vi "Control Panel Values Changed.vi"(8 "error in (no error)":errorcluster, 9 "Old data":variant, 10 "New data":variant, 11 "Device in":refnum<class "Cryo-Con-22C.lvclass">) -> (0 "error out":errorcluster, 3 "Device out":refnum<class "Cryo-Con-22C.lvclass">)   [LabVIEW 2015, in "Cryo-Con-22C.lvclass"]
uses:
  Cryo-Con-22C.lvclass
  Cryo-Con Front Panel Data.ctl
  Cryo-con Heater Ranges.ctl
  Cry-Con Loop Type.ctl
  Instrument/Read VISA Resource.vi
  Instrument/Write VISA Resource.vi
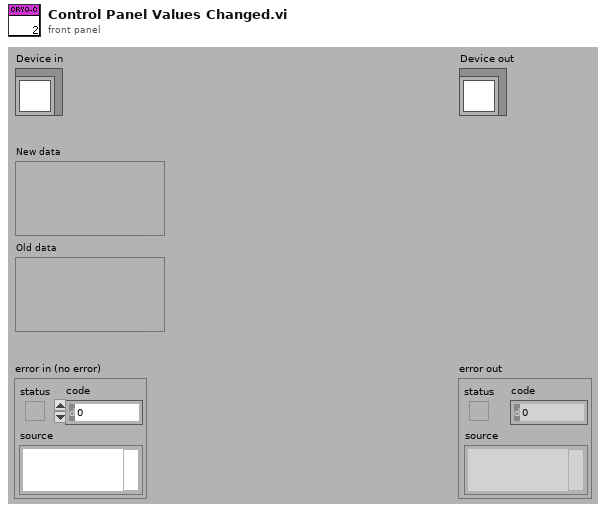
[diagram p1: front panel]
types:
  T1 = typedef "Cryo-Con Front Panel Data.ctl" = cluster{"Channels to measure":string[], "Record heater":bool, "Set point":dbl, "Heater Range":T2, "Control":bool, "Loop type":T3, "Ramp rate,\n K/min":dbl, "Control Channel":string, "P":dbl, "I":dbl, "D":dbl, "Manual %":u16}
  T2 = typedef "Cryo-con Heater Ranges.ctl" = enum16{"25W", "2.5W", "0.25W"}
  T3 = typedef "Cry-Con Loop Type.ctl" = enum16{"Off", "PID", "Manual", "PID Table", "PID Ramp", "PID Table Ramp"}
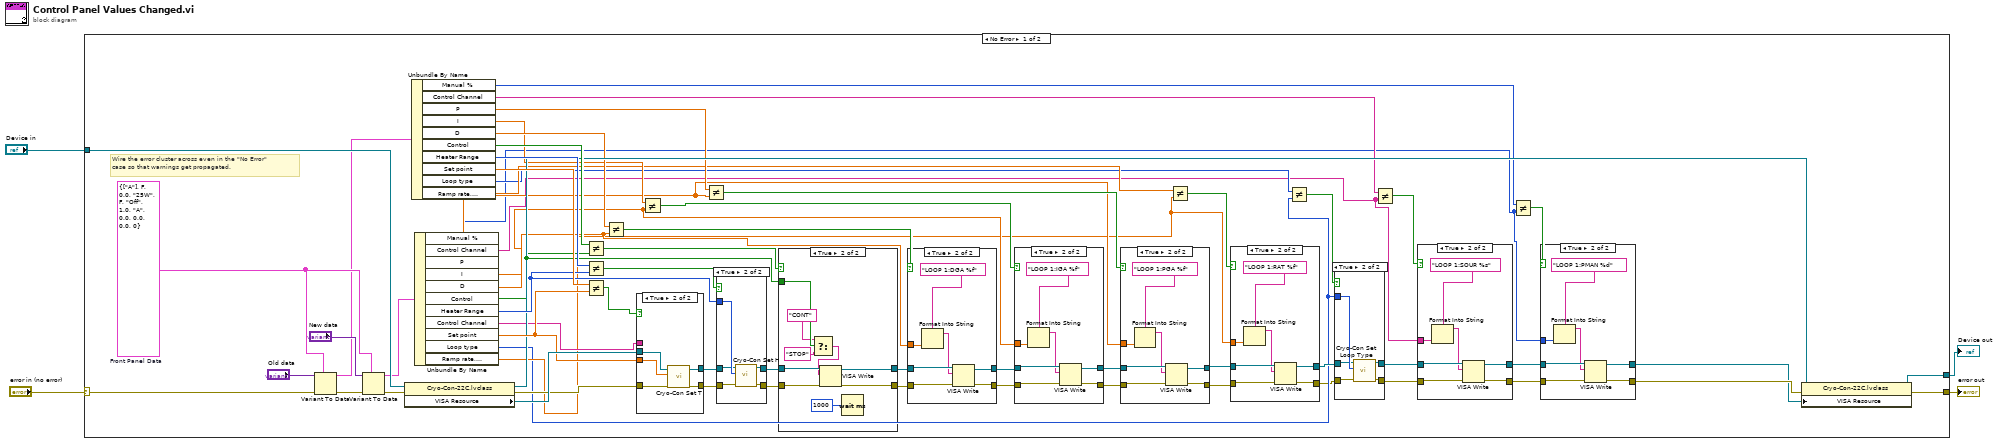
[diagram p0: block diagram]
diagram:
  n1 = case shown="No Error" "error in (no error)" {
    selector: "error in (no error)" -> [w69 w157]
    tunnel: [w66 w157] -> w3
    tunnel: [w67 w156] -> w1
    tunnel: "Device in" -> [w68 w156]
    frame No Error {
      w64 = T1 {"Channels to measure"=["A"], "Record heater"=FALSE, "Set point"=0.0, "Heater Range"=enum."25W", "Control"=FALSE, "Loop type"=enum."Off", "Ramp rate,\n K/min"=1.0, "Control Channel"="A", "P"=0.0, "I"=0.0, "D"=0.0, "Manual %"=0}  # Front Panel Data
      # "Wire the error cluster across even in the \"No Error\"\ncase so that warnings get propagated."
      n2 = Variant To Data(error in=w69, type=w64, Variant="Old data") -> (data=w44:T1, error out=w65:errorcluster)
      n3 = Variant To Data(error in=w65, type=w64, Variant="New data") -> (data=w45:T1, error out=w61:errorcluster)
      n4 = property class="Cryo-Con-22C.lvclass"(reference=w68, error in=w61) -> (reference out=w47:refnum<class "Cryo-Con-22C.lvclass">, error out=w60:errorcluster, "VISA Resource"=w62:refnum<visa-resource-name>)
      n5 = Unbundle By Name(w44) -> ("Manual %"=w11:u16, "Control Channel"=w16:string, "P"=w29:dbl, "I"=w35:dbl, "D"=w40:dbl, "Control"=w53:bool, "Heater Range"=w58:T2, "Set point"=w63:dbl, "Loop type"=w20:T3, "Ramp rate,\n K/min"=w26:dbl)
      n6 = Unbundle By Name(w45) -> ("Manual %"=w9:u16, "Control Channel"=w14:string, "P"=w28:dbl, "I"=w33:dbl, "D"=w38:dbl, "Control"=w41:bool, "Heater Range"=w48:T2, "Control Channel"=w46:string, "Set point"=w49:dbl, "Loop type"=w18:T3, "Ramp rate,\n K/min"=w24:dbl)
      n7 = Not Equal?(x=w53, y=w41) -> (x != y?=w55:bool)
      n8 = Not Equal?(x=w58, y=w48) -> (x != y?=w59:bool)
      n9 = Not Equal?(x=w63, y=w49) -> (x != y?=w27:bool)
      n10 = Not Equal?(x=w40, y=w38) -> (x != y?=w39:bool)
      n11 = case shown="True" w27 {
        tunnel: w60 -> [w150 w155]
        tunnel: [w150 w154] -> w57
        tunnel: w49 -> [_ w151]
        tunnel: w62 -> [w149 w152]
        tunnel: [w149 w153] -> w56
        tunnel: w46 -> [_ _]
        frame False {
        }
        frame True {
          n12 = call "Cryo-Con Set T.vi"("error in (no error)"=w155, "Set T"=w151, "VISA Resource Name"=w152) -> ("error out"=w154:errorcluster, "VISA Resource Name Out"=w153:refnum<visa-resource-name>)  [unwired: 7 in]
        }
      }
      n13 = Not Equal?(x=w35, y=w33) -> (x != y?=w34:bool)
      n14 = Not Equal?(x=w29, y=w28) -> (x != y?=w30:bool)
      n15 = case shown="True" w59 {
        tunnel: w57 -> [w143 w146]
        tunnel: [w143 w145] -> w54
        tunnel: w48 -> [_ w148]
        tunnel: [w142 w144] -> w52
        tunnel: w56 -> [w142 w147]
        frame False {
        }
        frame True {
          n16 = call "Cryo-Con Set H.vi"("error in (no error)"=w146, "Set T"=w148, "VISA Resource Name"=w147) -> ("error out"=w145:errorcluster, "VISA Resource Name Out"=w144:refnum<visa-resource-name>)  [unwired: 7 in]
        }
      }
      n17 = case shown="True" w55 {
        tunnel: w54 -> [w132 w139]
        tunnel: [w132 w141] -> w42
        tunnel: w41 -> [_ w137]
        tunnel: [w131 w138] -> w43
        tunnel: w52 -> [w131 w140]
        frame False {
        }
        frame True {
          n18 = Select(t="CONT", s=w137, f="STOP") -> (s? t:f=w134:string)
          n19 = VISA Write(VISA resource name=w140, write buffer=w134, error in (no error)=w139) -> (VISA resource name out=w138:refnum<visa-resource-name>, error out=w141:errorcluster)  [unwired: 1 out]
          n20 = Wait (ms)(milliseconds to wait=u32 1000) -> ()  [unwired: 1 out]
        }
      }
      n21 = case shown="True" w39 {
        tunnel: w42 -> [w123 w128]
        tunnel: [w123 w130] -> w36
        tunnel: w38 -> [_ w126]
        tunnel: [w122 w127] -> w37
        tunnel: w43 -> [w122 w129]
        frame False {
        }
        frame True {
          n22 = Format Into String(format string="LOOP 1:DGA %f", w126) -> (resulting string=w124:string)  [unwired: 2 in, 1 out]
          n23 = VISA Write(VISA resource name=w129, write buffer=w124, error in (no error)=w128) -> (VISA resource name out=w127:refnum<visa-resource-name>, error out=w130:errorcluster)  [unwired: 1 out]
        }
      }
      n24 = case shown="True" w34 {
        tunnel: w36 -> [w114 w119]
        tunnel: [w114 w121] -> w31
        tunnel: w33 -> [_ w117]
        tunnel: [w113 w118] -> w32
        tunnel: w37 -> [w113 w120]
        frame False {
        }
        frame True {
          n25 = Format Into String(format string="LOOP 1:IGA %f", w117) -> (resulting string=w115:string)  [unwired: 2 in, 1 out]
          n26 = VISA Write(VISA resource name=w120, write buffer=w115, error in (no error)=w119) -> (VISA resource name out=w118:refnum<visa-resource-name>, error out=w121:errorcluster)  [unwired: 1 out]
        }
      }
      n27 = case shown="True" w30 {
        tunnel: w31 -> [w105 w110]
        tunnel: [w105 w112] -> w23
        tunnel: w28 -> [_ w108]
        tunnel: [w104 w109] -> w22
        tunnel: w32 -> [w104 w111]
        frame False {
        }
        frame True {
          n28 = Format Into String(format string="LOOP 1:PGA %f", w108) -> (resulting string=w106:string)  [unwired: 2 in, 1 out]
          n29 = VISA Write(VISA resource name=w111, write buffer=w106, error in (no error)=w110) -> (VISA resource name out=w109:refnum<visa-resource-name>, error out=w112:errorcluster)  [unwired: 1 out]
        }
      }
      n30 = Not Equal?(x=w26, y=w24) -> (x != y?=w25:bool)
      n31 = case shown="True" w25 {
        tunnel: w23 -> [w96 w101]
        tunnel: [w96 w103] -> w17
        tunnel: w24 -> [_ w99]
        tunnel: [w95 w100] -> w21
        tunnel: w22 -> [w95 w102]
        frame False {
        }
        frame True {
          n32 = Format Into String(format string="LOOP 1:RAT %f", w99) -> (resulting string=w97:string)  [unwired: 2 in, 1 out]
          n33 = VISA Write(VISA resource name=w102, write buffer=w97, error in (no error)=w101) -> (VISA resource name out=w100:refnum<visa-resource-name>, error out=w103:errorcluster)  [unwired: 1 out]
        }
      }
      n34 = Not Equal?(x=w20, y=w18) -> (x != y?=w19:bool)
      n35 = case shown="True" w19 {
        tunnel: w17 -> [w89 w92]
        tunnel: [w89 w91] -> w12
        tunnel: w18 -> [_ w94]
        tunnel: [w88 w90] -> w13
        tunnel: w21 -> [w88 w93]
        frame False {
        }
        frame True {
          n36 = call "Cryo-Con Set Loop Type.vi"("error in (no error)"=w92, "Set T"=w94, "VISA Resource Name"=w93) -> ("error out"=w91:errorcluster, "VISA Resource Name Out"=w90:refnum<visa-resource-name>)  [unwired: 7 in]
        }
      }
      n37 = Not Equal?(x=w16, y=w14) -> (x != y?=w15:bool)
      n38 = case shown="True" w15 {
        tunnel: w12 -> [w80 w85]
        tunnel: [w80 w87] -> w8
        tunnel: w14 -> [_ w83]
        tunnel: [w79 w84] -> w7
        tunnel: w13 -> [w79 w86]
        frame False {
        }
        frame True {
          n39 = Format Into String(format string="LOOP 1:SOUR %s", w83) -> (resulting string=w81:string)  [unwired: 2 in, 1 out]
          n40 = VISA Write(VISA resource name=w86, write buffer=w81, error in (no error)=w85) -> (VISA resource name out=w84:refnum<visa-resource-name>, error out=w87:errorcluster)  [unwired: 1 out]
        }
      }
      n41 = Not Equal?(x=w11, y=w9) -> (x != y?=w10:bool)
      n42 = case shown="True" w10 {
        tunnel: w8 -> [w71 w76]
        tunnel: [w71 w78] -> w6
        tunnel: w9 -> [_ w74]
        tunnel: [w70 w75] -> w5
        tunnel: w7 -> [w70 w77]
        frame False {
        }
        frame True {
          n43 = Format Into String(format string="LOOP 1:PMAN %d", w74) -> (resulting string=w72:string)  [unwired: 2 in, 1 out]
          n44 = VISA Write(VISA resource name=w77, write buffer=w72, error in (no error)=w76) -> (VISA resource name out=w75:refnum<visa-resource-name>, error out=w78:errorcluster)  [unwired: 1 out]
        }
      }
      n45 = property class="Cryo-Con-22C.lvclass"(reference=w47, error in=w6, "VISA Resource"=w5) -> (reference out=w67:refnum<class "Cryo-Con-22C.lvclass">, error out=w66:errorcluster)
    }
    frame Error {
    }
  }
  "error out" <- w3
  "Device out" <- w1
